vi "Open Line Followers.vi"(8 "error in":errorcluster) -> (0 "error out":errorcluster)   [LabVIEW 2018]
uses:
  TypeDefs/typedef_enum_Refnums.ctl
  <vilib>/Rock Robotics/SystemInterfaces/DIO/FPGA_DIOChannel.ctl
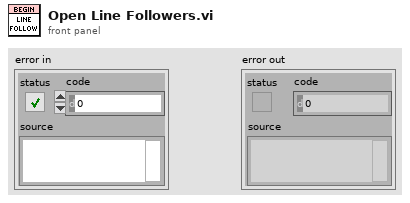
[diagram p1: front panel]
types:
  T1 = typedef "FPGA_DIOChannel.ctl" = enum8{"DIO 0", "DIO 1", "DIO 2", "DIO 3", "DIO 4", "DIO 5", "DIO 6", "DIO 7", "DIO 8", "DIO 9", "DIO MXP 0", "DIO MXP 1", "DIO MXP 2", "DIO MXP 3", "DIO MXP 4", "DIO MXP 5", "DIO MXP 6", "DIO MXP 7", "DIO MXP 8", "DIO MXP 9", "DIO MXP 10", "DIO MXP 11", "DIO MXP 12", "DIO MXP 13", "DIO MXP 14", "DIO MXP 15", "SPI Port CS1", "SPI Port CS2", "SPI Port CS3", "SPI Port MISO", "SPI Port MOSI", "Invalid"}
  T2 = typedef "typedef_enum_Refnums.ctl" = enum16{"Ball_Encoder", "Ball_Motor", "Camera", "Linefollow_3", "Linefollow_2", "Linefollow_1", "Gyro", "Hatch_Solenoid", "Climb_Back_Solenoid", "Arm_Encoder", "Arm_Motor", "Lift_Encoder", "Drive", "Drive_Motor_R", "Drive_Motor_L", "Drive_Encoder_R", "Drive_Encoder_L", "Joy_R", "Joy_L", "Wrist_Motor", "Wrist_Encoder", "Climb Upper Limit", "Climb Lower Limit ", "Climb_Front_Motor"}
  T3 = typedef "WPI_DigitalInputDevRef.ctl" = cluster{"DevStatus":errorcluster, "DIO Channel":T1}
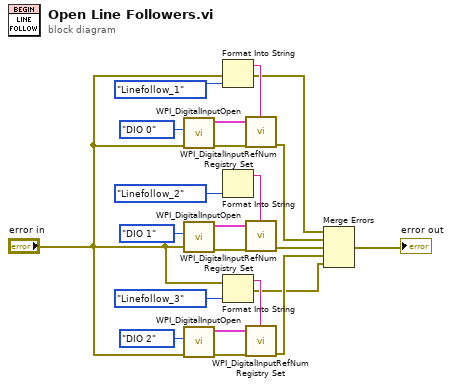
[diagram p0: block diagram]
diagram:
  n1 = call <vilib>:"WPI_DigitalInputOpen.vi"("error in (no error)"="error in", "DIO Channel"=FPGA_DIOChannel."DIO 0") -> ("error out"=w22:errorcluster, "DigitalInputDevRef"=w21:T3)  [unwired: 8 in]
  n2 = call <vilib>:"WPI_DigitalInputOpen.vi"("error in (no error)"="error in", "DIO Channel"=FPGA_DIOChannel."DIO 1") -> ("error out"=w18:errorcluster, "DigitalInputDevRef"=w17:T3)  [unwired: 8 in]
  n3 = call <vilib>:"WPI_DigitalInputOpen.vi"("error in (no error)"="error in", "DIO Channel"=FPGA_DIOChannel."DIO 2") -> ("error out"=w14:errorcluster, "DigitalInputDevRef"=w13:T3)  [unwired: 8 in]
  n4 = Format Into String(error in="error in", typedef_enum_Refnums."Linefollow_1" ("RefNums")) -> (resulting string=w20:string, error out=w1:errorcluster)  [unwired: 2 in]
  n5 = Format Into String(typedef_enum_Refnums."Linefollow_2" ("RefNums")) -> (resulting string=w16:string)  [unwired: 3 in, 1 out]
  n6 = Format Into String(error in="error in", typedef_enum_Refnums."Linefollow_3" ("RefNums")) -> (resulting string=w12:string, error out=w3:errorcluster)  [unwired: 2 in]
  n7 = call <vilib>:"WPI_DigitalInputRefNum Registry Set.vi"("error in (no error)"=w22, "refnum name"=w20, "DigitalInputDevRef"=w21) -> ("error out"=w9:errorcluster)  [unwired: 7 in, 1 out]
  n8 = call <vilib>:"WPI_DigitalInputRefNum Registry Set.vi"("error in (no error)"=w18, "refnum name"=w16, "DigitalInputDevRef"=w17) -> ("error out"=w10:errorcluster)  [unwired: 7 in, 1 out]
  n9 = call <vilib>:"WPI_DigitalInputRefNum Registry Set.vi"("error in (no error)"=w14, "refnum name"=w12, "DigitalInputDevRef"=w13) -> ("error out"=w8:errorcluster)  [unwired: 7 in, 1 out]
  n10 = Merge Errors(w1, w9, w10, w8, w3) -> (→"error out":errorcluster)
